vi "DELETE_snapshot_item_from_db.vi"(10 "SnapID":string, 11 "API Key":string="cheia04042025tema2restfulapi") -> (3 "DELETE_clear_specific_error_header":string)   [LabVIEW 2024]
uses:
  <vilib>/httpClient/LabVIEWHTTPClient.lvlib
panel:
  out "delete_error_":string
  out "error out delete error memory":errorcluster
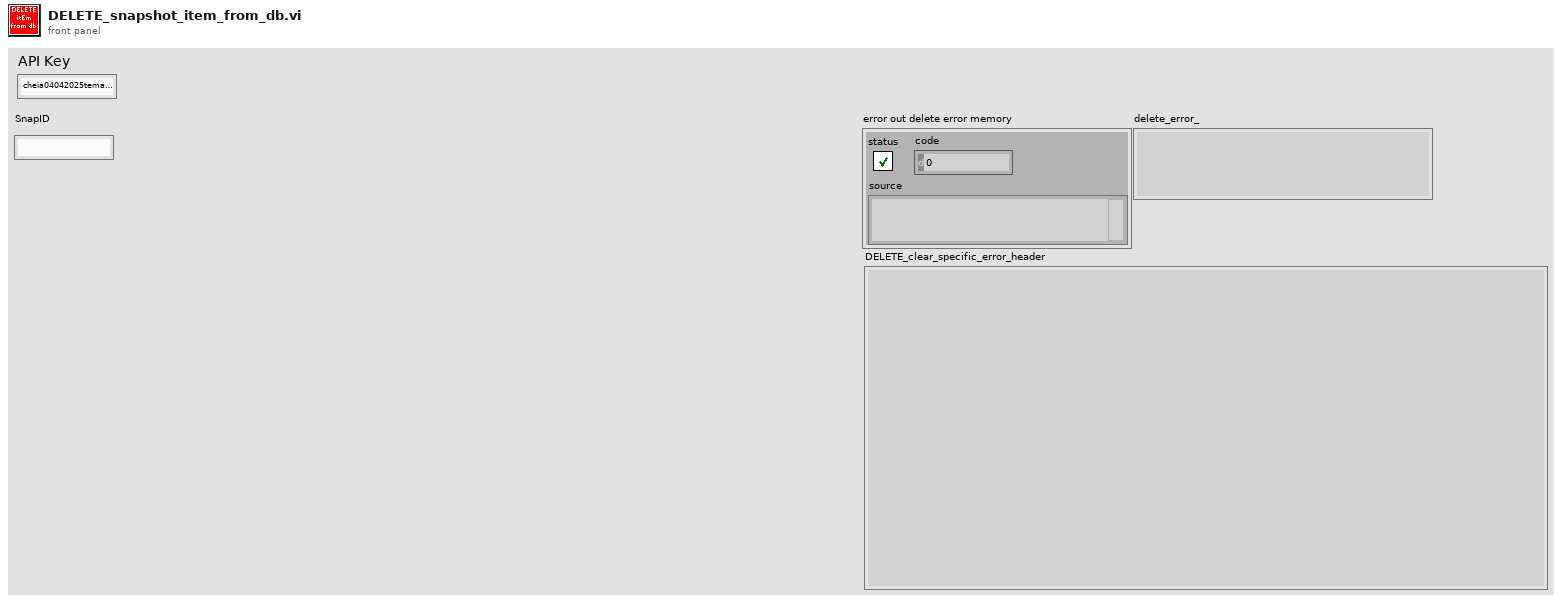
[diagram p1: front panel]
types:
  T1 = typedef "LabVIEWHTTPClient.lvlib/ClientHandle.ctl" = refnum<k1>
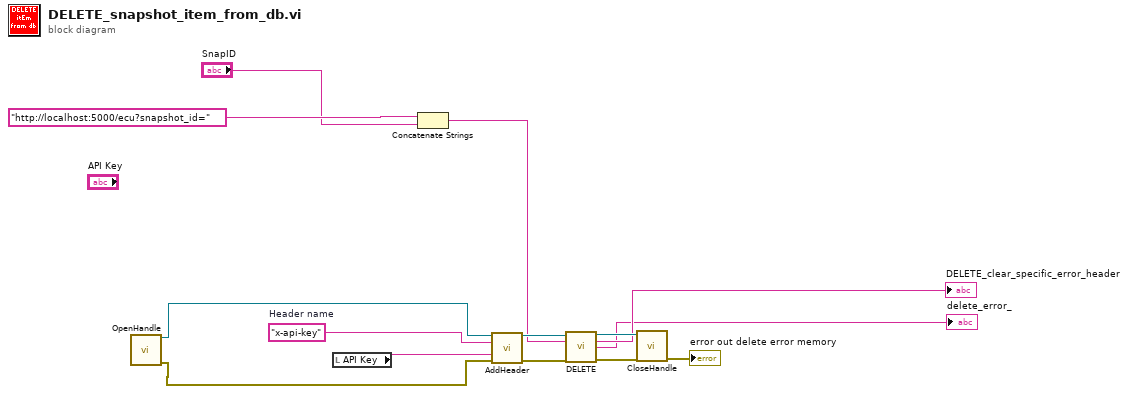
[diagram p0: block diagram]
diagram:
  w7 = "x-api-key"  # Header name
  n1 = call <vilib>:"OpenHandle.vi"() -> ("client handle out"=w8:T1, "error out"=w9:errorcluster)  [unwired: 14 in]
  n2 = local read "API Key"() -> (w6:string)
  n3 = Concatenate Strings("http://localhost:5000/ecu?snapshot_id=" ("url"), "SnapID") -> (w2:string)
  n4 = call <vilib>:"AddHeader.vi"("client handle"=w8, "header"=w7, "value"=w6, "error in (no error)"=w9) -> ("client handle out"=w11:T1, "error out"=w10:errorcluster)  [unwired: 10 in]
  n5 = call <vilib>:"DELETE.vi"("client handle"=w11, "url"=w2, "error in (no error)"=w10) -> ("client handle out"=w13:T1, "headers"=→"DELETE_clear_specific_error_header":string, "body"=→"delete_error_":string, "error out"=w12:errorcluster)  [unwired: 9 in]
  n6 = call <vilib>:"CloseHandle.vi"("client handle"=w13, "error in (no error)"=w12) -> ("error out"=→"error out delete error memory":errorcluster)  [unwired: 13 in]
